vi "fgv_manual-auto.vi"(7 "cmd":enum16{"write", "read"}(ring), 8 "error in":errorcluster, 11 "manual":bool) -> (0 "error out":errorcluster, 3 "manual check":bool)   [LabVIEW 2019]
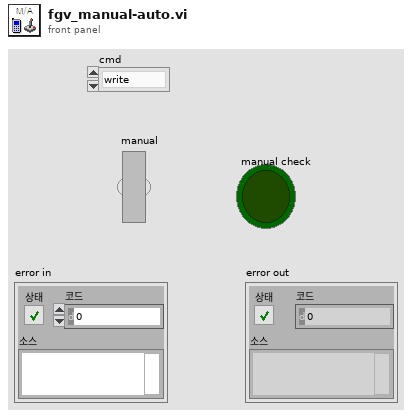
[diagram p1: front panel]
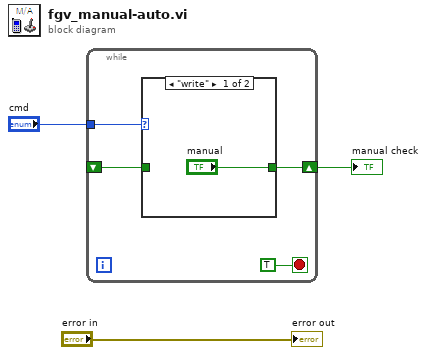
[diagram p0: block diagram]
diagram:
  n1 = while {
    tunnel: "cmd" -> [w6]
    shift-right: [w5] -> w2
    shift-left: _ -> [w4]
    stop <- TRUE stop-if-true
    n2 = case shown="\"write\"" w6 {
      tunnel: ["manual" w9] -> w5
      tunnel: w4 -> [_ w9]
      frame "write" {
      }
      frame "read", Default {
      }
    }
  }
  "manual check" <- w2
  "error out" <- "error in"
